vi "moveSCUTest.vi"   [LabVIEW 2013, in "main.lvlib"]
uses:
  main.lvlib
types:
  T1 = cluster{"port":i32, "AEtitle":string, "host":string, "remoteAE":string}
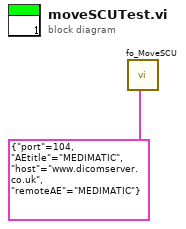
[diagram p0: block diagram]
diagram:
  n1 = call "fo_MoveSCU.vi"("ServerInfo"=T1 {"port"=104, "AEtitle"="MEDIMATIC", "host"="www.dicomserver.co.uk", "remoteAE"="MEDIMATIC"}) -> ()  [unwired: 10 in, 1 out]
